vi "ParameterParser.vi"(2 "Parameter String":string) -> (0 "Remaining Parameter String":string, 1 "Parameter":dbl)   [LabVIEW 2019]
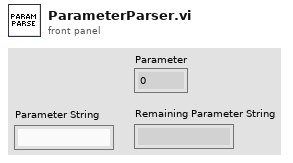
[diagram p1: front panel]
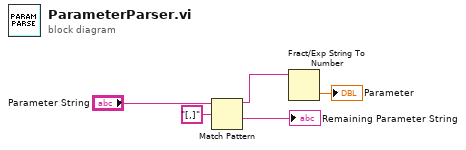
[diagram p0: block diagram]
diagram:
  n1 = Match Pattern(string="Parameter String", regular expression="[,]") -> (before substring=w2:string, after substring=→"Remaining Parameter String":string)  [unwired: 1 in, 2 out]
  n2 = Fract/Exp String To Number(string=w2) -> (number=→"Parameter":dbl)  [unwired: 3 in, 1 out]
